vi "Begin UI Update.vi"(8 "Error In":errorcluster, 11 "State In":T1) -> (0 "Error Out":errorcluster, 3 "State Out":T1)   [LabVIEW 2017, in "Eulogy.lvlib" / "Bookmark Manager.lvlib"]
uses:
  Bookmark Manager.lvlib
  State.ctl
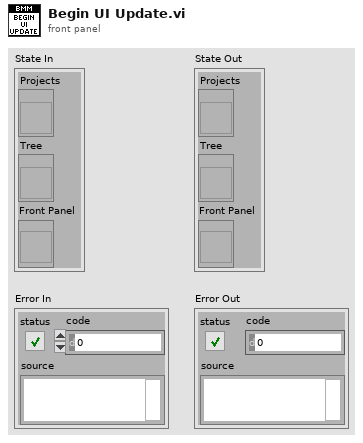
[diagram p1: front panel]
types:
  T1 = typedef "Eulogy.lvlib/Bookmark Manager.lvlib/State.ctl" = cluster{"Projects":refnum<vi>, "Tree":refnum<vi>, "Front Panel":refnum<vi>}
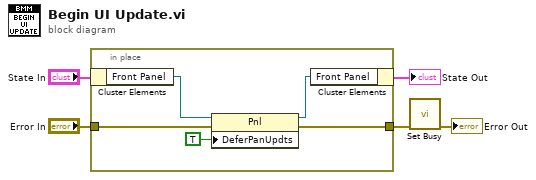
[diagram p0: block diagram]
diagram:
  n1 = in-place {
    in-place-border: "Error In" -> [w7]
    in-place-border: [w6] -> w5
    n2 = in-place-cluster #1("State In") -> ("Front Panel"=w10:refnum<vi>)
    n3 = property class="Pnl"(reference=w10, error in=w7, "DeferPanUpdts"=TRUE ("Defer Panel Updates")) -> (reference out=w9:refnum<vi>, error out=w6:errorcluster)
    n4 = in-place-cluster #1("Front Panel"=w9) -> (→"State Out":T1)
  }
  n5 = call <vilib>:"Set Busy.vi"("error in (no error)"=w5) -> ("error out"=→"Error Out":errorcluster)  [unwired: 9 in, 1 out]
